vi "ArrayMax.vi"(9 "Array":dbl[](array[numeric])) -> (1 "max":dbl)   [LabVIEW 2016]
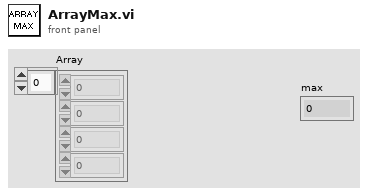
[diagram p1: front panel]
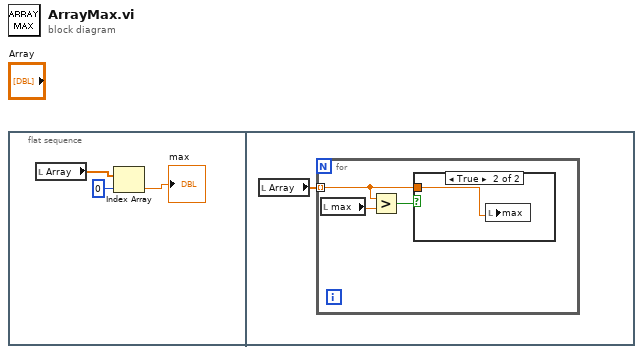
[diagram p0: block diagram]
diagram:
  n1 = flat-sequence {
    frame #0 {
      n2 = local read "Array"() -> (w2:dbl[])
      n3 = Index Array(array=w2, index=0) -> (element=→"max":dbl)
    }
    frame #1 {
      n4 = local read "Array"() -> (w4:dbl[])
      n5 = for {
        tunnel: w4 -> [w6] mode=indexing
        n6 = local read "max"() -> (w7:dbl)
        n7 = Greater?(x=w6, y=w7) -> (0:w5:bool)
        n8 = case shown="True" w5 {
          tunnel: w6 -> [_ w8]
          frame False {
          }
          frame True {
            n9 = local write "max"(w8) -> ()
          }
        }
      }
    }
  }
